vi "Initialize Configuration.vi"(8 "error in (no error)":errorcluster, 11 "Instrument in":refnum<class "Instrument.lvclass">) -> (0 "error out":errorcluster, 3 "Instrument out":refnum<class "Instrument.lvclass">)   [LabVIEW 2019, in "Instrument.lvclass"]
uses:
  Instrument.lvclass
  Instrument.lvclass/Instrument.ctl
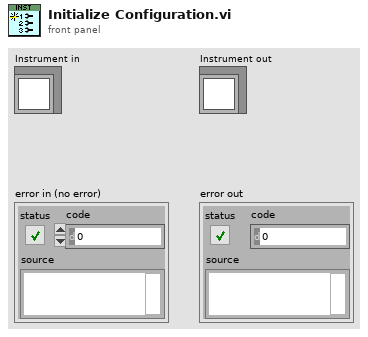
[diagram p1: front panel]
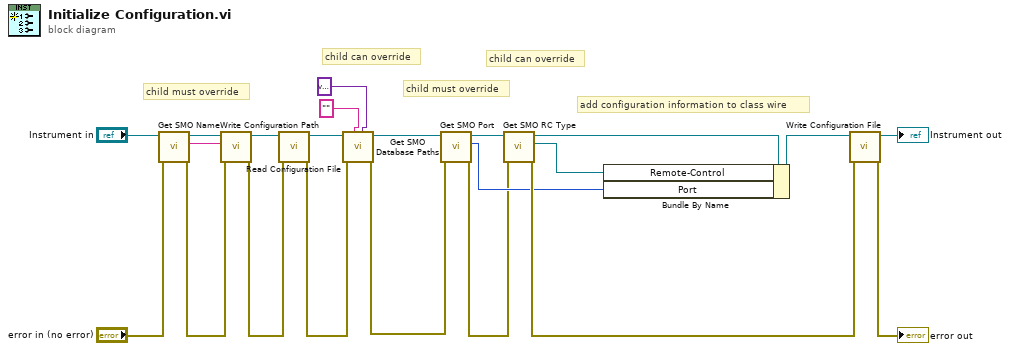
[diagram p0: block diagram]
diagram:
  # "child can override"
  # "child can override"
  # "child must override"
  # "child must override"
  # "add configuration information to class wire"
  n1 = call-dynamic "Get SMO Name.vi"("error in (no error)"="error in (no error)", "Instrument in"="Instrument in") -> ("error out"=w7:errorcluster, "SMO Name"=w18:string, "Instrument out"=w8:refnum<class "Instrument.lvclass">)  [unwired: 7 in]
  n2 = call "Write Configuration Path.vi"("error in (no error)"=w7, "name or relative path"=w18, "Instrument in"=w8) -> ("error out"=w14:errorcluster, "Instrument out"=w13:refnum<class "Instrument.lvclass">)  [unwired: 7 in]
  n3 = call-dynamic "Read Configuration File.vi"("error in (no error)"=w14, "Instrument in"=w13) -> ("error out"=w1:errorcluster, "Instrument out"=w15:refnum<class "Instrument.lvclass">)  [unwired: 8 in]
  n4 = call-dynamic "Get SMO Database Paths.vi"("getAll Cluster"=variant, "Default Paths"="", "error in (no error)"=w1, "Instrument in"=w15) -> ("error out"=w17:errorcluster, "Instrument out"=w16:refnum<class "Instrument.lvclass">)  [unwired: 5 in, 1 out]
  n5 = call-dynamic "Get SMO Port.vi"("error in (no error)"=w17, "Instrument in"=w16) -> ("error out"=w10:errorcluster, "Port"=w11:u16, "Instrument out"=w9:refnum<class "Instrument.lvclass">)  [unwired: 7 in]
  n6 = call-dynamic "Get SMO RC Type.vi"("error in (no error)"=w10, "Instrument in"=w9) -> ("error out"=w20:errorcluster, "RemoteControl"=w4:refnum<class "RemoteControl.lvclass">, "Instrument out"=w12:refnum<class "Instrument.lvclass">)  [unwired: 7 in]
  n7 = Bundle By Name(cluster=w12, "Remote-Control"=w4, "Port"=w11) -> (w22:refnum<class "Instrument.lvclass">)
  n8 = call-dynamic "Write Configuration File.vi"("error in (no error)"=w20, "Instrument in"=w22) -> ("error out"=→"error out":errorcluster, "Instrument out"=→"Instrument out":refnum<class "Instrument.lvclass">)  [unwired: 8 in]
